vi "Example Custom Row Cell Types.vi"() -> ()   [LabVIEW 2013]
doc: "This examples shows off many of the basic usage patterns of the datagrid."
uses:
  GridColumn/ColumnDefinition.ctl
  GridColumn/ColumnType.ctl
  DataGridView/DataGridView.lvclass
  DataGridView/DataGridView.lvclass/DataGridView.ctl
  DataGridView/Properties/Read registeredEvents.vi
  DataGridView/Properties/Read DataGridView.vi
  Events/Abstract EVENT/Abstract EVENT.lvclass
  DataGrid.lvlib
  Events/KeyDown/KeyDown.lvclass
  System.Windows.Forms
  Events/CellDirtyStateChanged/CellDirtyStateChanged.lvclass
  Events/CellValueChanged/CellValueChanged.lvclass
  GridColumn/GridColumn.lvclass
panel:
  out "cell value 2":string
  out "cell value":string
  in  "Cells":T2(array[cluster])=[[{"datatype"=enum."string", "Value"="Test", "Params"=""}, {"datatype"=enum."string", "Value"="All my details here.", "Params"=""}, {"datatype"=enum."timestamp", "Value"="2015-11-25 8:48 AM", "Params"=""}, {"datatype"=enum."combo", "Value"="PL", "Params"="PT|PL|UT|Probe"}, {"datatype"=enum."button", "Value"="Test", "Params"=""}, {"datatype"=enum."numeric", "Value"="12.4", "Params"=""}, {"datatype"=enum."image", "Value"="16_released.png", "Params"=""}, {"datatype"=enum."check", "Value"="True", "Params"=""}, {"datatype"=enum."link", "Value"="http://ni.com", "Params"=""}], [{"datatype"=enum."numeric", "Value"="33", "Params"=""}, {"datatype"=enum."check", "Value"="T", "Params"=""}, {"datatype"=enum."link", "Value"="http://Learnthis.ca", "Params"=""}, {"datatype"=enum."image", "Value"="16_info.png", "Params"=""}, {"datatype"=enum."combo", "Value"="B", "Params"="A|B|C"}, {"datatype"=enum."combo", "Value"="PL", "Params"="PL|PT|TR|SR"}, {"datatype"=enum."combo", "Value"="GUAGE", "Params"="GUAGE|TEST|DATA"}, {"datatype"=enum."string", "Value"="none", "Params"=""}, {"datatype"=enum."string", "Value"="anything", "Params"=""}]]
  in  "ColumnSetup":T3[](array[typedef])=[{"name"="Text", "caption"="", "datatype"=enum."string", "Params"="", "AutoSizeMode"=2, "FillWeight"=15.0, "MinWidth"=40, "tooltip"=""}, {"name"="Details", "caption"="", "datatype"=enum."string", "Params"="", "AutoSizeMode"=16, "FillWeight"=100.0, "MinWidth"=150, "tooltip"=""}, {"name"="Time", "caption"="", "datatype"=enum."string", "Params"="", "AutoSizeMode"=1, "FillWeight"=1.0, "MinWidth"=140, "tooltip"=""}, {"name"="Combo", "caption"="", "datatype"=enum."string", "Params"="One|Two|Three", "AutoSizeMode"=6, "FillWeight"=1.0, "MinWidth"=80, "tooltip"=""}, {"name"="Function", "caption"="", "datatype"=enum."string", "Params"="", "AutoSizeMode"=6, "FillWeight"=1.0, "MinWidth"=50, "tooltip"=""}, {"name"="Value", "caption"="", "datatype"=enum."string", "Params"="", "AutoSizeMode"=6, "FillWeight"=1.0, "MinWidth"=10, "tooltip"=""}, {"name"="Active", "caption"="", "datatype"=enum."string", "Params"="", "AutoSizeMode"=6, "FillWeight"=1.0, "MinWidth"=10, "tooltip"=""}, {"name"="Status", "caption"="", "datatype"=enum."string", "Params"="", "AutoSizeMode"=6, "FillWeight"=1.0, "MinWidth"=10, "tooltip"=""}, {"name"="Link", "caption"="", "datatype"=enum."string", "Params"="", "AutoSizeMode"=1, "FillWeight"=100.0, "MinWidth"=50, "tooltip"=""}] {"MinWidth" min=2 step=1; "AutoSizeMode" items=["None"=1, "ColumnHeader"=2, "AllCellsExceptHeader"=4, "AllCells"=6, "DisplayedCellsExceptHeader"=8, "DisplayedCells"=10, "Fill"=16]; "FillWeight" min=1 max=100}
  in  "DataGridView":refnum<k24>(container)
  # "INSTRUCTIONS:\n1. ColumnSetup defines the columns \n2. Use Cells to override the column types \n3. Run the VI, interactions will show as events"
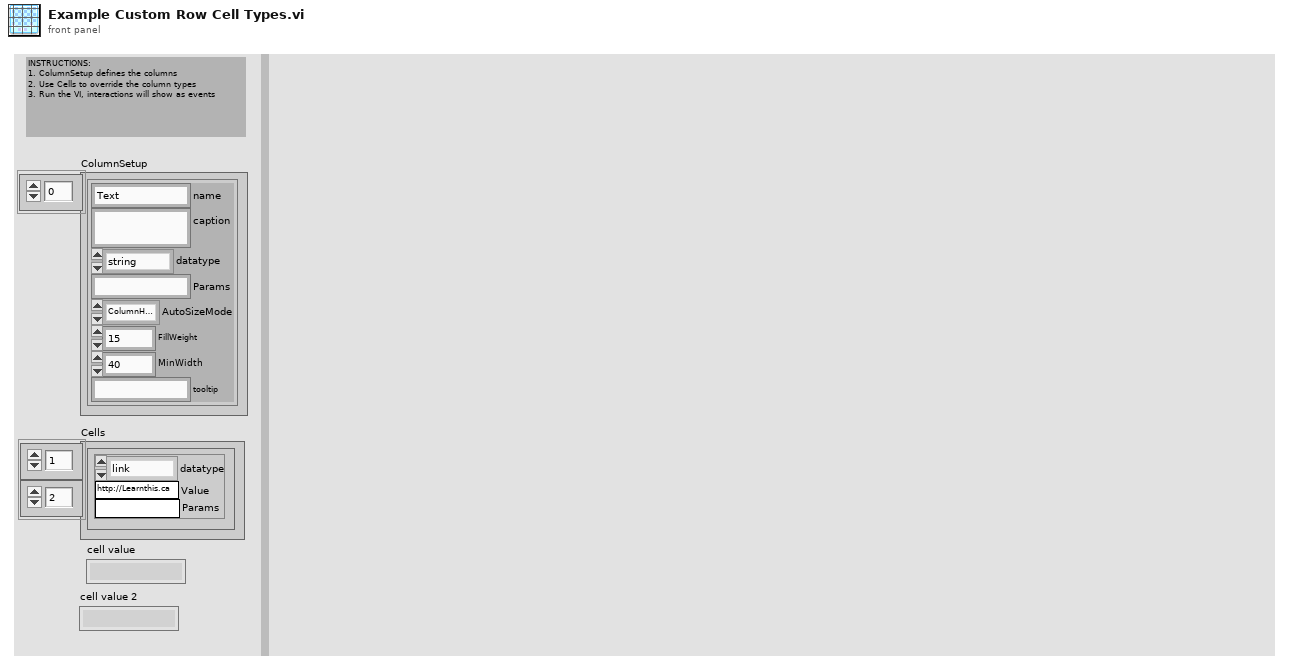
[diagram p1: front panel]
types:
  T1 = typedef "DataGrid.lvlib/GridColumn.lvclass/ColumnType.ctl" = enum16{"string", "image", "check", "numeric", "timestamp", "button", "combo", "link"}
  T2 = cluster{"datatype":T1, "Value":string, "Params":string}[][]
  T3 = typedef "DataGrid.lvlib/GridColumn.lvclass/ColumnDefinition.ctl" = cluster{"name":string, "caption":string, "datatype":T1, "Params":string, "AutoSizeMode":i32, "FillWeight":sgl, "MinWidth":u32, "tooltip":string}
  T4 = cluster{"Alt":bool, "Control":bool, "KeyCode":i32, "KeyData":i32, "KeyValue":i32, "Modifiers":i32, "Shift":bool}
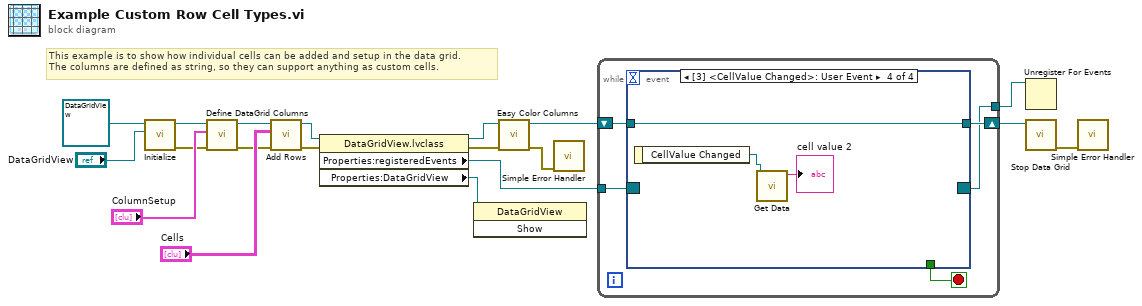
[diagram p0: block diagram]
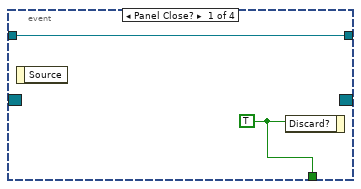
[diagram p2: hidden frame]
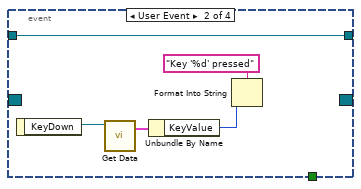
[diagram p3: hidden frame]
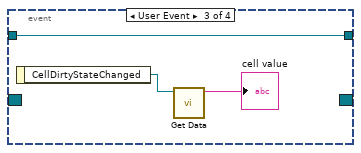
[diagram p4: hidden frame]
diagram:
  # "This example is to show how individual cells can be added and setup in the data grid.\nThe columns are defined as string, so they can support anything as custom cells."
  n1 = call "Initialize.vi"("DataGridView"="DataGridView", "DataGrid in"=refnum<class "DataGridView.lvclass"> refnum) -> ("error out"=w4:errorcluster, "DataGrid out"=w8:refnum<class "DataGridView.lvclass">)  [unwired: 8 in]
  n2 = call "Define DataGrid Columns.vi"("error in (no error)"=w4, "ColumnSetup"="ColumnSetup", "DataGrid in"=w8) -> ("error out"=w5:errorcluster, "DataGrid out"=w7:refnum<class "DataGridView.lvclass">)  [unwired: 6 in, 1 out]
  n3 = call "Add Rows.vi"("error in (no error)"=w5, "Cells"="Cells", "DataGridView in"=w7) -> ("error out"=w2:errorcluster, "DataGridView out"=w3:refnum<class "DataGridView.lvclass">)  [unwired: 7 in]
  n4 = property class="DataGridView.lvclass"(reference=w3, error in=w2) -> (reference out=w12:refnum<class "DataGridView.lvclass">, error out=w13:errorcluster, "Properties:registeredEvents"=w11:refnum<event-registration>, "Properties:DataGridView"=w1:refnum<k24>)
  n5 = invoke class="DataGridView" method="Show"(reference=w1) -> ()  [unwired: 2 in, 3 out]
  n6 = call "Easy Color Columns.vi"("error in (no error)"=w13, "DataGridView in"=w12) -> ("error out"=w19:errorcluster, "DataGridView out"=w18:refnum<class "DataGridView.lvclass">)  [unwired: 8 in]
  n7 = call <vilib>:"Simple Error Handler.vi"("error in (no error)"=w19) -> ()  [unwired: 4 in, 5 out]
  n8 = while {
    tunnel: w11 -> [w23]
    shift-right: [w21] -> w17
    shift-left: w18 -> [w22]
    tunnel: [w20] -> w16
    stop <- w24 stop-if-true
    n9 = event shown="[3] <CellValue Changed>: User Event" {
      selector: w23 -> [_ _ _ _]
      dyn-events: [_ _ _ _] -> w20
      timeout: _ -> [_ _ _ _]
      tunnel: [w26 _ _ _] -> w24
      tunnel: w22 -> [w25 w31 w34 w37]
      tunnel: [w25 w31 w34 w37] -> w21
      event Panel Close? {
        w26 = TRUE ("Discard?")
        n10 = event-data() -> ()  [unwired: 1 in, 1 out]
        n11 = event-data("Discard?"=w26) -> ()  [unwired: 1 in, 1 out]
      }
      event User Event {
        n12 = event-data() -> ("KeyDown"=w30:refnum<class "Abstract EVENT.lvclass">)  [unwired: 1 in]
        n13 = call "Get Data.vi"("DataGrid.lvlib:Abstract EVENT.lvclass"=w30) -> ("output cluster"=w28:T4)  [unwired: 9 in, 1 out]
        n14 = Unbundle By Name(w28) -> ("KeyValue"=w27:i32)
        n15 = Format Into String(format string="Key '%d' pressed" ("message"), w27) -> ()  [unwired: 2 in, 2 out]
      }
      event User Event {
        n16 = event-data() -> ("CellDirtyStateChanged"=w32:refnum<class "Abstract EVENT.lvclass">)  [unwired: 1 in]
        n17 = call "Get Data.vi"("DataGrid.lvlib:Abstract EVENT.lvclass"=w32) -> ("cell value"=→"cell value":string)  [unwired: 7 in, 3 out]
      }
      event User Event {
        n18 = event-data() -> ("CellValue Changed"=w36:refnum<class "Abstract EVENT.lvclass">)  [unwired: 1 in]
        n19 = call "Get Data.vi"("DataGrid.lvlib:Abstract EVENT.lvclass"=w36) -> ("cell value"=→"cell value 2":string)  [unwired: 7 in, 3 out]
      }
    }
  }
  n20 = Unregister For Events(event registration refnum=w16) -> ()  [unwired: 1 in, 1 out]
  n21 = call "Stop Data Grid.vi"("DataGridView in"=w17) -> ("error out"=w15:errorcluster)  [unwired: 9 in, 1 out]
  n22 = call <vilib>:"Simple Error Handler.vi"("error in (no error)"=w15) -> ()  [unwired: 4 in, 5 out]
